vi "SAVETOUCH.vi"   [LabVIEW 2016, in "Test2.lvrbt"]
uses:
  Test2.lvrbt
  <vilib>/NXT/Block Support/NXT_InputPort.ctl
  <vilib>/NXT/Hardware/Plugins/Tetrix DC Motor/TetrixDCMotorAddress.ctl
  <vilib>/NXT/Hardware/Plugins/Tetrix 180 deg Servo/Tetrix180ServoAddress.ctl
  <vilib>/NXT/NXTIO Xnodes/NXTIONodeSubVIs/TETRIX IO Move Servos.vi
  <vilib>/NXT/Dual Mode Library/Waits/Wait_Num.vi
  <vilib>/NXT/NXTIO Xnodes/NXTIONodeSubVIs/TETRIX IO Move DC Motors.vi
  <vilib>/NXT/Dual Mode Library/Waits/Wait_EV3_Ultrasonic_Centimeter_Closer.vi
  <vilib>/NXT/NXTIO Xnodes/NXTIONodeSubVIs/TETRIX IO Stop DC Motors.vi
  <vilib>/NXT/Dual Mode Library/Waits/Wait_EV3_Ultrasonic_Centimeters_Further.vi
  <vilib>/NXT/Dual Mode Library/Waits/Wait_Touch.vi
  <vilib>/NXT/NXTIO Xnodes/AddressXNode/NXTIOAddress.xnode
  <vilib>/NXT/Subs/LVHSConnector.ctl
  <vilib>/NXT/NXTIO Xnodes/NXTIOXNode/NXTIO.xnode
  <vilib>/NXT/LegoClasses/BrickReference/BrickReference.lvclass
types:
  T1 = typedef "NXT_InputPort.ctl" = u32
  T2 = typedef "Tetrix180ServoAddress.ctl" = i32
  T3 = cluster{"Tetrix180Servo":T2, "Tetrix180Servo":T2, "Tetrix180Servo":T2, "Tetrix180Servo":T2, "Tetrix180Servo":T2, "Tetrix180Servo":T2}
  T4 = typedef "TetrixDCMotorAddress.ctl" = i32
  T5 = typedef "LVHSConnector.ctl" = refnum<class "BrickReference.lvclass">
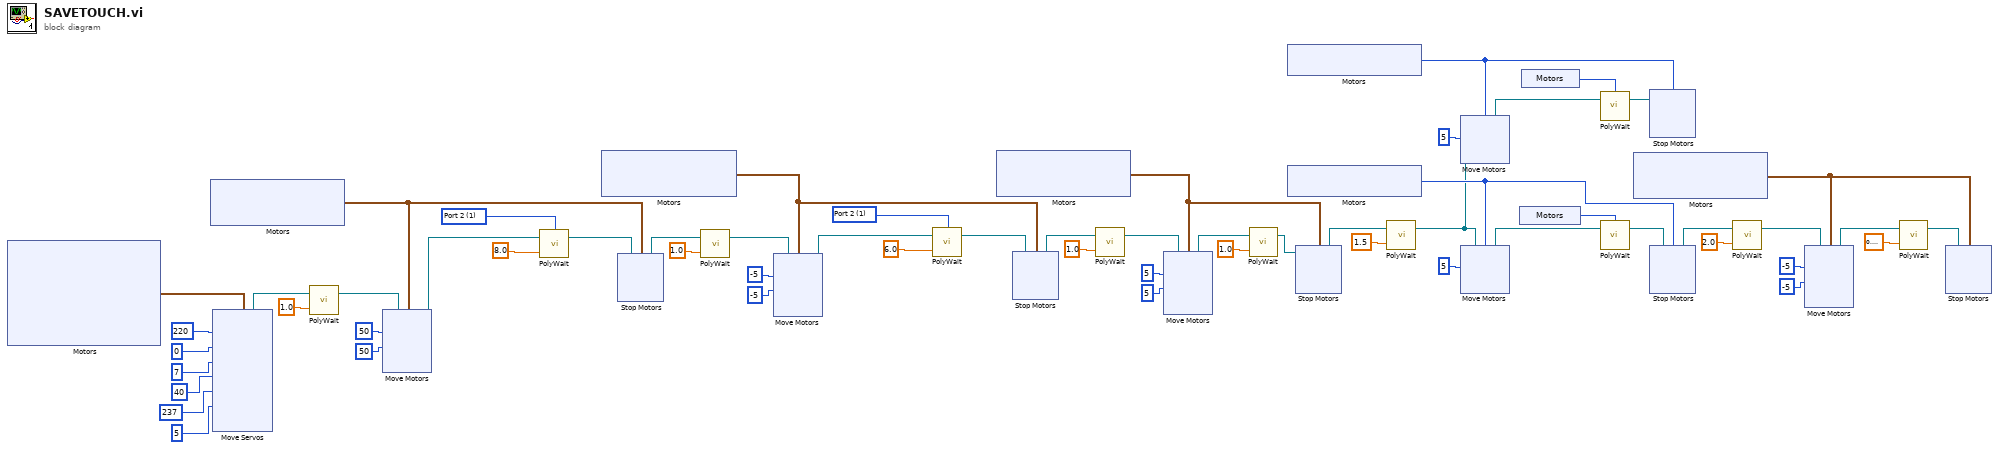
[diagram p0: block diagram]
diagram:
  w13 = T1 1 items=["Port 1", "Port 2", "Port 3", "Port 4"] ("Port (Port 1)")
  w40 = T1 1 items=["Port 1", "Port 2", "Port 3", "Port 4"] ("Port (Port 1)")
  n1 = xnode "Motors"() -> ("Motor"=w29:T3)
  n2 = xnode "Motors"() -> ("Motor"=w53:cluster{"TetrixDCMotor":T4, "TetrixDCMotor":T4})
  n3 = xnode "Move Servos"("Position 6"=u8 5, "Position 5"=u8 237, "Position 4"=u8 40, "Position 3"=u8 7, "Position 2"=u8 0, "Position 1"=u8 220, "Motors"=w29) -> ("NXT/EV3"=w22:T5)  [unwired: 1 in]
  n4 = call-poly <vilib>:"PolyWait.vi"("Time (1 sec)"=sgl 1.0, "NXT/EV3"=w22) -> ("NXT/EV3"=w21:T5)  [unwired: 2 in]
  n5 = xnode "Move Motors"("Power/Speed 2"=i8 50, "Power/Speed 1"=i8 50, "Motors"=w53, "NXT/EV3"=w21) -> ("NXT/EV3"=w56:T5)
  n6 = call-poly <vilib>:"PolyWait.vi"("Centimeters (40)"=sgl 8.0, "NXT/EV3"=w56, "Port (Port 1)"=w40) -> ("NXT/EV3"=w54:T5)  [unwired: 1 in]
  n7 = xnode "Motors"() -> ("Motor"=w10:cluster{"TetrixDCMotor":T4, "TetrixDCMotor":T4})
  n8 = xnode "Stop Motors"("Motors"=w53, "NXT/EV3"=w54) -> ("NXT/EV3"=w19:T5)
  n9 = call-poly <vilib>:"PolyWait.vi"("Time (1 sec)"=sgl 1.0, "NXT/EV3"=w19) -> ("NXT/EV3"=w2:T5)  [unwired: 2 in]
  n10 = xnode "Move Motors"("Power/Speed 2"=i8 -5, "Power/Speed 1"=i8 -5, "Motors"=w10, "NXT/EV3"=w2) -> ("NXT/EV3"=w16:T5)
  n11 = call-poly <vilib>:"PolyWait.vi"("Centimeters (50)"=sgl 6.0, "NXT/EV3"=w16, "Port (Port 1)"=w13) -> ("NXT/EV3"=w14:T5)  [unwired: 1 in]
  n12 = xnode "Motors"() -> ("Motor"=w4:cluster{"TetrixDCMotor":T4, "TetrixDCMotor":T4})
  n13 = xnode "Stop Motors"("Motors"=w10, "NXT/EV3"=w14) -> ("NXT/EV3"=w8:T5)
  n14 = call-poly <vilib>:"PolyWait.vi"("Time (1 sec)"=sgl 1.0, "NXT/EV3"=w8) -> ("NXT/EV3"=w7:T5)  [unwired: 2 in]
  n15 = xnode "Move Motors"("Power/Speed 2"=i8 5, "Power/Speed 1"=i8 5, "Motors"=w4, "NXT/EV3"=w7) -> ("NXT/EV3"=w6:T5)
  n16 = call-poly <vilib>:"PolyWait.vi"("Time (1 sec)"=sgl 1.0, "NXT/EV3"=w6) -> ("NXT/EV3"=w5:T5)  [unwired: 2 in]
  n17 = xnode "Motors"() -> ("Motor"=w49:T4)
  n18 = xnode "Motors"() -> ("Motor"=w45:T4)
  n19 = xnode "Stop Motors"("Motors"=w4, "NXT/EV3"=w5) -> ("NXT/EV3"=w1:T5)
  n20 = call-poly <vilib>:"PolyWait.vi"("Time (1 sec)"=sgl 1.5, "NXT/EV3"=w1) -> ("NXT/EV3"=w43:T5)  [unwired: 2 in]
  n21 = xnode "Move Motors"("Power/Speed 1"=i8 5, "Motors"=w49, "NXT/EV3"=w43) -> ("NXT/EV3"=w51:T5)
  n22 = xnode "Move Motors"("Power/Speed 1"=i8 5, "Motors"=w45, "NXT/EV3"=w43) -> ("NXT/EV3"=w46:T5)
  n23 = xnode "Motors"() -> ("Sensor"=w42:T1)
  n24 = xnode "Motors"() -> ("Sensor"=w41:T1)
  n25 = call-poly <vilib>:"PolyWait.vi"("NXT/EV3"=w51, "Port (Port 1)"=w41) -> ("NXT/EV3"=w50:T5)  [unwired: 2 in]
  n26 = call-poly <vilib>:"PolyWait.vi"("NXT/EV3"=w46, "Port (Port 1)"=w42) -> ("NXT/EV3"=w44:T5)  [unwired: 2 in]
  n27 = xnode "Motors"() -> ("Motor"=w37:cluster{"TetrixDCMotor":T4, "TetrixDCMotor":T4})
  n28 = xnode "Stop Motors"("Motors"=w49, "NXT/EV3"=w50) -> ()  [unwired: 1 out]
  n29 = xnode "Stop Motors"("Motors"=w45, "NXT/EV3"=w44) -> ("NXT/EV3"=w39:T5)
  n30 = call-poly <vilib>:"PolyWait.vi"("Time (1 sec)"=sgl 2.0, "NXT/EV3"=w39) -> ("NXT/EV3"=w35:T5)  [unwired: 2 in]
  n31 = xnode "Move Motors"("Power/Speed 2"=i8 -5, "Power/Speed 1"=i8 -5, "Motors"=w37, "NXT/EV3"=w35) -> ("NXT/EV3"=w32:T5)
  n32 = call-poly <vilib>:"PolyWait.vi"("Time (1 sec)"=sgl 0.2, "NXT/EV3"=w32) -> ("NXT/EV3"=w31:T5)  [unwired: 2 in]
  n33 = xnode "Stop Motors"("Motors"=w37, "NXT/EV3"=w31) -> ()  [unwired: 1 out]
